vi "_Set Default.vi"   [LabVIEW 2015]
uses:
  <vilib>/rvi/eio/common/nirviEmuTemplateMethod_errors.vi
  <vilib>/eio/EIONode/EIONode.xnode
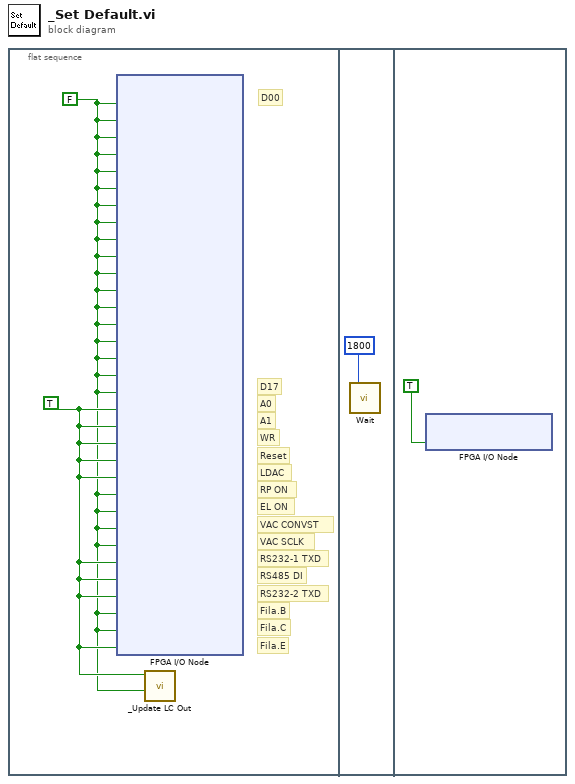
[diagram p0: block diagram]
diagram:
  n1 = flat-sequence {
    frame #0 {
      w2 = TRUE
      w1 = FALSE ("Port4/DIO8")
      # "RS232-2 TXD"
      # "RS485 DI"
      # "RS232-1 TXD"
      # "Fila.E"
      # "Fila.C"
      # "Fila.B"
      # "VAC SCLK"
      # "VAC CONVST"
      # "EL ON"
      # "RP ON"
      # "LDAC"
      # "WR"
      # "A1"
      # "A0"
      # "Reset"
      # "D17"
      # "D00"
      n2 = xnode "FPGA I/O Node"("Digtal IO/DIO42"=w1, "Digtal IO/DIO41"=w1, "Digtal IO/DIO40"=w1, "Digtal IO/DIO39"=w1, "Digtal IO/DIO38"=w1, "Digtal IO/DIO37"=w1, "Digtal IO/DIO36"=w1, "Digtal IO/DIO35"=w1, "Digtal IO/DIO34"=w1, "Digtal IO/DIO32"=w1, "Digtal IO/DIO31"=w1, "Digtal IO/DIO30"=w1, "Digtal IO/DIO29"=w1, "Digtal IO/DIO28"=w1, "Digtal IO/DIO27"=w1, "Digtal IO/DIO26"=w1, "Digtal IO/DIO25"=w1, "Digtal IO/DIO24"=w1, "Digtal IO/DIO62"=w2, "Digtal IO/DIO61"=w2, "Digtal IO/DIO64"=w2, "Digtal IO/DIO13"=w2, "Digtal IO/DIO63"=w2, "Digtal IO/DIO18"=w1, "Digtal IO/DIO23"=w1, "Digtal IO/DIO57"=w1, "Digtal IO/DIO58"=w1, "Digtal IO/DIO45"=w2, "Digtal IO/DIO47"=w2, "Digtal IO/DIO55"=w2, "Digtal IO/DIO66"=w1, "Digtal IO/DIO67"=w1, "Digtal IO/DIO68"=w2) -> ()  [unwired: 33 in, 33 out]
      n3 = call "_Update LC Out.vi"("LC Stop"=w1, "LC Hold"=w2) -> ()  [unwired: 6 out]
    }
    frame #1 {
      n4 = call "Wait"("Count(mSec)"=u16 1800) -> ()  [unwired: 1 out]
    }
    frame #2 {
      n5 = xnode "FPGA I/O Node"("Digtal IO/DIO57"=TRUE ("Port4/DIO8")) -> ()  [unwired: 1 in, 1 out]
    }
  }
